vi "Lab2_2.vi"() -> ()   [LabVIEW 2017]
panel:
  out "Sine":dbl(graph)
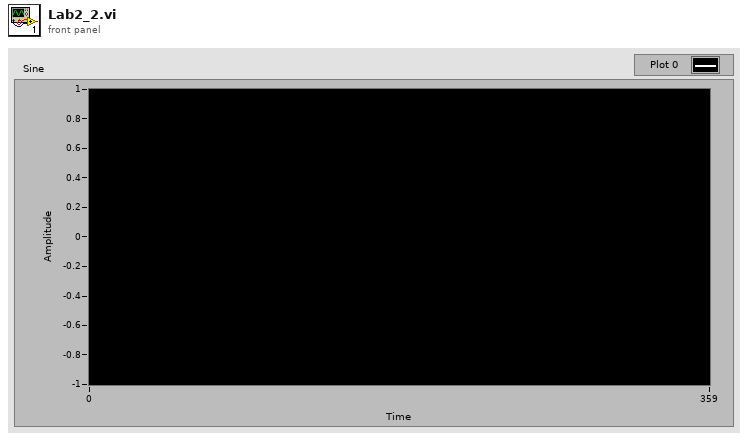
[diagram p1: front panel]
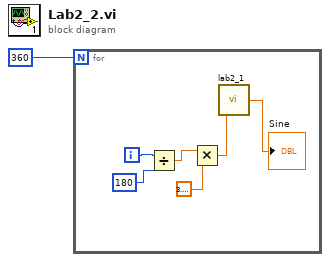
[diagram p0: block diagram]
diagram:
  n1 = for {
    N: 360 -> [_]
    i -> [w7]
    n2 = Divide(x=w7, y=180) -> (x/y=w5:dbl)
    n3 = Multiply(x=w5, y=3.141592653589793) -> (x*y=w3:dbl)
    n4 = call "lab2_1.vi"("x"=w3) -> ("sin(x)"=→"Sine":dbl)
  }
